vi "run all.vi"(8 "error in":errorcluster, 11 "vi modification tool in":refnum<class "VI modification collection.lvclass">) -> (0 "error report":errorcluster[](array[cluster]), 3 "vi modification tool out":refnum<class "VI modification collection.lvclass">)   [LabVIEW 2013, in "VI modification collection.lvclass"]
uses:
  VI modification collection.lvclass
  VI modification collection.lvclass/VI modification collection.ctl
  VI modification.lvclass/VI modification.ctl
  VI modification.lvclass
  Read exclusions.vi
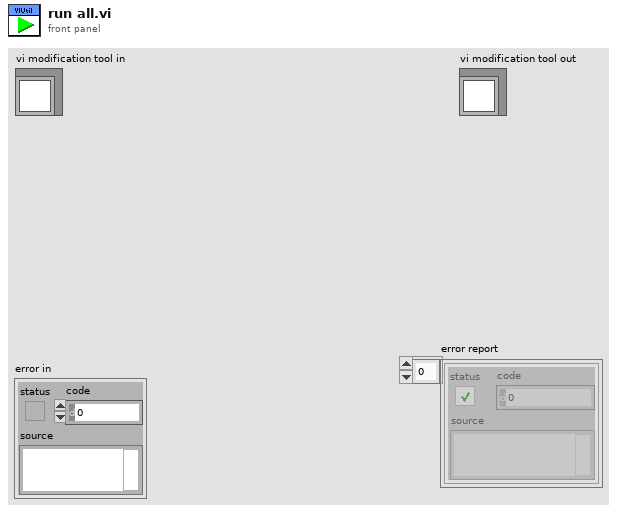
[diagram p1: front panel]
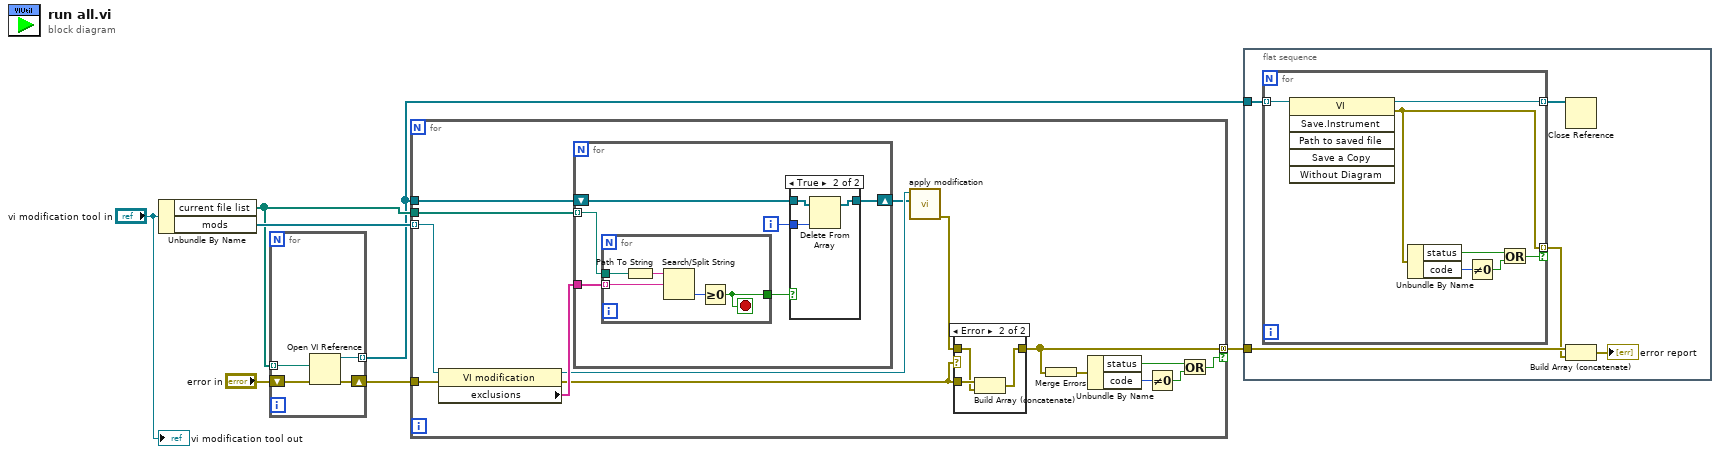
[diagram p0: block diagram]
diagram:
  n1 = Unbundle By Name("vi modification tool in") -> ("current file list"=w2:path[], "mods"=w6:refnum<class "VI modification.lvclass">[])
  n2 = for {
    shift-right: [w9] -> w3
    shift-left: "error in" -> [w11]
    tunnel: w2 -> [w10] mode=indexing
    tunnel: [w8] -> w1 mode=indexing
    n3 = Open VI Reference(vi path=w10, error in (no error)=w11) -> (vi reference=w8:refnum<vi>, error out=w9:errorcluster)  [unwired: 4 in]
  }
  n4 = for {
    tunnel: w6 -> [w17] mode=indexing
    tunnel: w3 -> [w26]
    tunnel: [w24] -> w5 mode=concatenating if=w20
    tunnel: w2 -> [w25]
    tunnel: w1 -> [w19]
    n5 = property class="VI modification"(reference=w17, error in=w26) -> (reference out=w15:refnum<class "VI modification.lvclass">, error out=w12:errorcluster, "exclusions"=w16:string[])
    n6 = for {
      tunnel: w25 -> [w36] mode=indexing
      tunnel: w16 -> [w35]
      shift-right: [w32] -> w14
      shift-left: w19 -> [w33]
      i -> [w31]
      n7 = for {
        tunnel: w36 -> [w41]
        tunnel: w35 -> [w45] mode=indexing
        tunnel: [w43] -> w34
        stop <- w43 stop-if-true
        n8 = Path To String(path=w41) -> (string=w42:string)
        n9 = Search/Split String(string=w42, search string/char (-)=w45) -> (offset of match=w44:i32)  [unwired: 1 in, 2 out]
        n10 = Greater Or Equal To 0?(x=w44) -> (x >= 0?=w43:bool)
      }
      n11 = case shown="True" w34 {
        tunnel: w33 -> [w37 w40]
        tunnel: [w37 w39] -> w32
        tunnel: w31 -> [_ w38]
        frame False {
        }
        frame True {
          n12 = Delete From Array(array=w40, index=w38) -> (array with subset deleted=w39:refnum<vi>[])  [unwired: 1 in, 1 out]
        }
      }
    }
    n13 = call-dynamic "apply modification.vi"("vis"=w14, "VI modification in"=w15) -> ("error report"=w13:errorcluster[])  [unwired: 8 in, 1 out]
    n14 = case shown="Error" w12 {
      tunnel: w12 -> [_ w30]
      tunnel: w13 -> [w27 w29]
      tunnel: [w27 w28] -> w24
      frame No Error {
      }
      frame Error {
        n15 = Build Array (concatenate)(w30, w29) -> (w28:errorcluster[])
      }
    }
    n16 = Merge Errors(w24) -> (w18:errorcluster)
    n17 = Unbundle By Name(w18) -> ("status"=w23:bool, "code"=w22:i32)
    n18 = Not Equal To 0?(x=w22) -> (x != 0?=w21:bool)
    n19 = Or(x=w23, y=w21) -> (x .or. y?=w20:bool)
  }
  n20 = flat-sequence {
    tunnel: w5 -> [w50]
    tunnel: w1 -> [w49]
    frame #0 {
      n21 = for {
        tunnel: w49 -> [w57] mode=indexing
        tunnel: [w56] -> w48 mode=indexing
        tunnel: [w51] -> w46 mode=indexing if=w52
        n22 = invoke class="VI" method="Save.Instrument"(reference=w57) -> (reference out=w56:refnum<vi>, error out=w51:errorcluster)  [unwired: 5 in, 4 out]
        n23 = Unbundle By Name(w51) -> ("status"=w53:bool, "code"=w54:i32)
        n24 = Not Equal To 0?(x=w54) -> (x != 0?=w55:bool)
        n25 = Or(x=w53, y=w55) -> (x .or. y?=w52:bool)
      }
      n26 = Close Reference(reference=w48) -> ()  [unwired: 1 in, 1 out]
      n27 = Build Array (concatenate)(w50, w46) -> (→"error report":errorcluster[])
    }
  }
  "vi modification tool out" <- "vi modification tool in"
